vi "Placeholder --error.vi"(10 "Error":errorcluster) -> (2 "Error":errorcluster)   [LabVIEW 2020, in "jettl.lvlib" / "Error.lvlib"]
uses:
  Error.lvlib
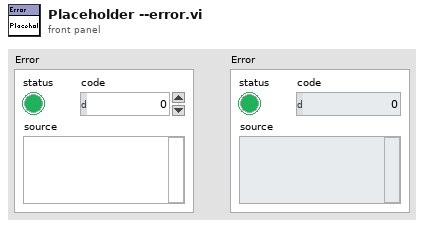
[diagram p1: front panel]
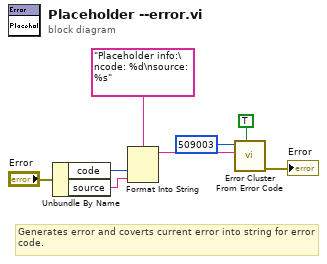
[diagram p0: block diagram]
diagram:
  # "Generates error and coverts current error into string for error code."
  n1 = Unbundle By Name("Error") -> ("code"=w2:i32, "source"=w1:string)
  n2 = Format Into String(format string="Placeholder info:\ncode: %d\nsource: %s", w2, w1) -> (resulting string=w5:string)  [unwired: 2 in, 1 out]
  n3 = call <vilib>:"Error Cluster From Error Code.vi"("show call chain? (False)"=TRUE, "error message (\"\")"=w5, "error code (0)"=509003) -> ("error out"=→"Error":errorcluster)  [unwired: 6 in]
